vi "Noise (G3)-Create.vi"(0 "Noise In":T1, 5 "Sampling Rate (Hz)":dbl, 7 "Npts":i32, 9 "Rep":i32, 11 "error in (no error)":errorcluster, 12 "Name":string) -> (4 "Noise Out":T1, 6 "Waveform":dbl[](array[numeric]), 15 "error out":errorcluster)   [LabVIEW 2020]
uses:
  Noise (G3).ctl
  Noise (G3).Properties.ctl
  Noise (G3).Data.ctl
  Waveform VIs/Noise VIs/Noise-Globals.vi
  <vilib>/Analysis/NI_AALBase.lvlib
  4th Generation/Classes/Filter/Filter.lvclass
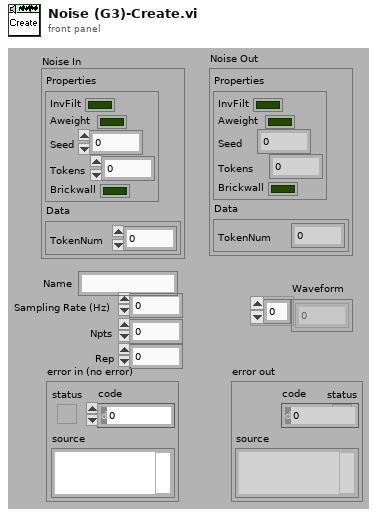
[diagram p1: front panel]
types:
  T1 = typedef "Noise (G3).ctl" = cluster{"Properties":T2, "Data":T3}
  T2 = typedef "Noise (G3).Properties.ctl" = cluster{"InvFilt":bool, "Aweight":bool, "Seed":i32, "Tokens":i32, "Brickwall":bool}
  T3 = typedef "Noise (G3).Data.ctl" = cluster{"TokenNum":i32}
  T4 = enum16{"Clear", "Set data", "Reset index", "Get data"}
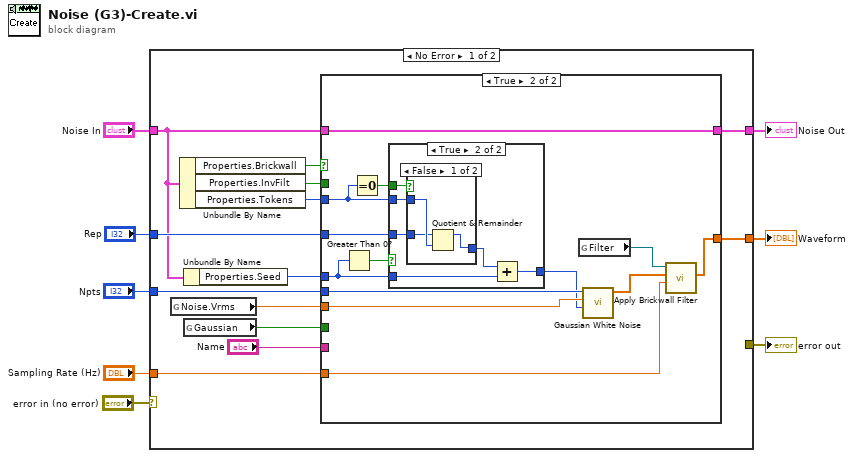
[diagram p0: block diagram]
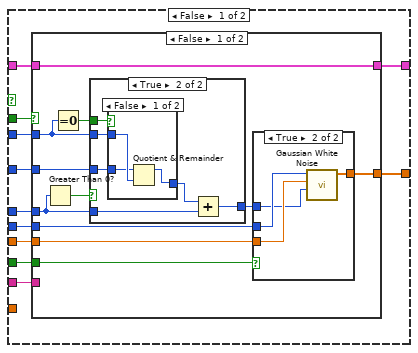
[diagram p2: hidden frame]
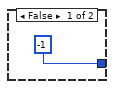
[diagram p3: hidden frame]
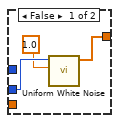
[diagram p5: hidden frame]
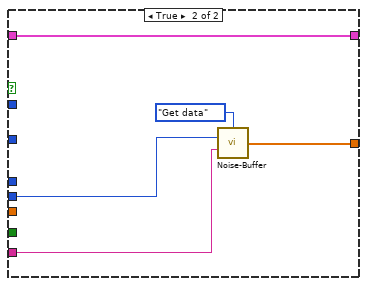
[diagram p6: hidden frame]
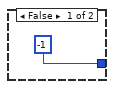
[diagram p7: hidden frame]
diagram:
  n1 = case shown="No Error" "error in (no error)" {
    selector: "error in (no error)" -> [_ w92]
    tunnel: "Npts" -> [w21 _]
    tunnel: [w20 _] -> w7
    tunnel: [_ w92] -> w5
    tunnel: [w19 w91] -> w3
    tunnel: "Noise In" -> [w13 w91]
    tunnel: "Rep" -> [w15 _]
    tunnel: "Sampling Rate (Hz)" -> [w9 _]
    frame No Error {
      n2 = global read "Noise-Globals.vi" "Noise.Vrms"() -> (w10:dbl)
      n3 = Unbundle By Name(w13) -> ("Properties.Brickwall"=w11:bool, "Properties.InvFilt"=w17:bool, "Properties.Tokens"=w14:i32)
      n4 = Unbundle By Name(w13) -> ("Properties.Seed"=w12:i32)
      n5 = global read "Noise-Globals.vi" "Gaussian"() -> (w18:bool)
      n6 = case shown="True" w11 {
        tunnel: w21 -> [w32 w77]
        tunnel: [w31 w74] -> w20
        tunnel: [w30 w79] -> w19
        tunnel: w18 -> [w29 _]
        tunnel: w10 -> [w28 w78]
        tunnel: w17 -> [w27 _]
        tunnel: "Name" -> [w26 _]
        tunnel: w15 -> [w25 w69]
        tunnel: w14 -> [w24 w70]
        tunnel: w13 -> [w23 w79]
        tunnel: w12 -> [w22 w67]
        tunnel: w9 -> [_ w76]
        frame False {
          n7 = case shown="False" w27 {
            tunnel: w32 -> [w43 w65]
            tunnel: [w42 w66] -> w31
            tunnel: w23 -> [w41 w62]
            tunnel: [w41 w62] -> w30
            tunnel: w29 -> [w40 _]
            tunnel: w28 -> [w39 _]
            tunnel: w26 -> [_ w64]
            tunnel: w25 -> [w38 _]
            tunnel: w24 -> [w34 _]
            tunnel: w22 -> [w36 _]
            frame False {
              n8 = Greater Than 0?(x=w36) -> (x > 0?=w35:bool)
              n9 = Equal To 0?(x=w34) -> (x = 0?=w33:bool)
              n10 = case shown="True" w35 {
                tunnel: w38 -> [_ w46]
                tunnel: w34 -> [_ w50]
                tunnel: w36 -> [_ w49]
                tunnel: [-1 w48] -> w37
                tunnel: w33 -> [_ w45]
                frame False {
                }
                frame True {
                  n11 = case shown="False" w45 {
                    tunnel: w50 -> [w53 _]
                    tunnel: [w52 w54] -> w47
                    tunnel: w46 -> [w51 w54]
                    frame False {
                      n12 = Quotient & Remainder(x=w51, y=w53) -> (x-y*floor(x/y)=w52:i32)  [unwired: 1 out]
                    }
                    frame True {
                    }
                  }
                  n13 = Add(x=w47, y=w49) -> (x+y=w48:i32)
                }
              }
              n14 = case shown="True" w40 {
                tunnel: w43 -> [w57 w60]
                tunnel: [w56 w61] -> w42
                tunnel: w39 -> [_ w59]
                tunnel: w37 -> [_ w58]
                frame False {
                  n15 = call <vilib>:"Uniform White Noise.vi"("amplitude"=1.0, "samples"=w57) -> ("uniform white noise"=w56:dbl[])  [unwired: 8 in, 1 out]
                }
                frame True {
                  n16 = call <vilib>:"Gaussian White Noise.vi"("seed"=w58, "standard deviation"=w59, "samples"=w60) -> ("Gaussian noise pattern"=w61:dbl[])  [unwired: 7 in, 1 out]
                }
              }
            }
            frame True {
              n17 = call "Noise-Buffer.vi"("Action"=T4."Get data", "Npts"=w65, "Name"=w64) -> ("Data Out"=w66:dbl[])  [unwired: 11 in, 1 out]
            }
          }
        }
        frame True {
          n18 = Greater Than 0?(x=w67) -> (x > 0?=w72:bool)
          n19 = Equal To 0?(x=w70) -> (x = 0?=w71:bool)
          n20 = case shown="True" w72 {
            tunnel: w69 -> [_ w82]
            tunnel: w70 -> [_ w86]
            tunnel: w67 -> [_ w85]
            tunnel: [-1 w84] -> w68
            tunnel: w71 -> [_ w81]
            frame False {
            }
            frame True {
              n21 = case shown="False" w81 {
                tunnel: w86 -> [w89 _]
                tunnel: [w88 w90] -> w83
                tunnel: w82 -> [w87 w90]
                frame False {
                  n22 = Quotient & Remainder(x=w87, y=w89) -> (x-y*floor(x/y)=w88:i32)  [unwired: 1 out]
                }
                frame True {
                }
              }
              n23 = Add(x=w83, y=w85) -> (x+y=w84:i32)
            }
          }
          n24 = global read "Noise-Globals.vi" "Filter"() -> (w73:refnum<class "Filter.lvclass">)
          n25 = call <vilib>:"Gaussian White Noise.vi"("seed"=w68, "standard deviation"=w78, "samples"=w77) -> ("Gaussian noise pattern"=w75:dbl[])  [unwired: 7 in, 1 out]
          n26 = call "Apply Brickwall Filter.vi"("Fs (Hz)"=w76, "Signal In"=w75, "Filter in"=w73) -> ("Signal Out"=w74:dbl[])  [unwired: 5 in, 3 out]
        }
      }
    }
    frame Error {
    }
  }
  "error out" <- w5
  "Waveform" <- w7
  "Noise Out" <- w3
